vi "Draw 2D Plot.vi"(6 "Control Ref Queue":T1, 8 "error in (no error)":errorcluster, 10 "Multiplot Representation In":T2, 11 "2D Compass.lvclass in":refnum<class "2D Compass.lvclass">) -> (0 "error out":errorcluster, 2 "Multiplot Representation Out":T2, 3 "2D Compass.lvclass out":refnum<class "2D Compass.lvclass">)   [LabVIEW 2017, in "2D Compass.lvclass"]
uses:
  <vilib>/Math Plots/2D Math Plots/2D Compass/2D Compass/2D Compass.lvclass
  <vilib>/Math Plots/2D Math Plots/2D Plot/2D Plot/Typedef/Multiplot Representation.ctl
  <vilib>/Math Plots/2D Math Plots/2D Plot/2D Plot/Typedef/Plot Representation.ctl
  <vilib>/Math Plots/2D Math Plots/2D Plot/2D Plot/Typedef/Range Cluster.ctl
  <vilib>/Math Plots/2D Math Plots/2D Plot/Action String/2DMathPlot Ctrl Act Queue.ctl
  <vilib>/Math Plots/2D Math Plots/2D Plot/Action String/2DMathPlot Ctrl Act Cluster.ctl
  <vilib>/Math Plots/2D Math Plots/2D Plot/Action String/2DMathPlot State Class.ctl
  <vilib>/Math Plots/2D Math Plots/2D Compass/2D Compass/2D Compass.lvclass/2D Compass.ctl
  <vilib>/Math Plots/2D Math Plots/2D Plot/2D Plot/2D Plot.lvclass
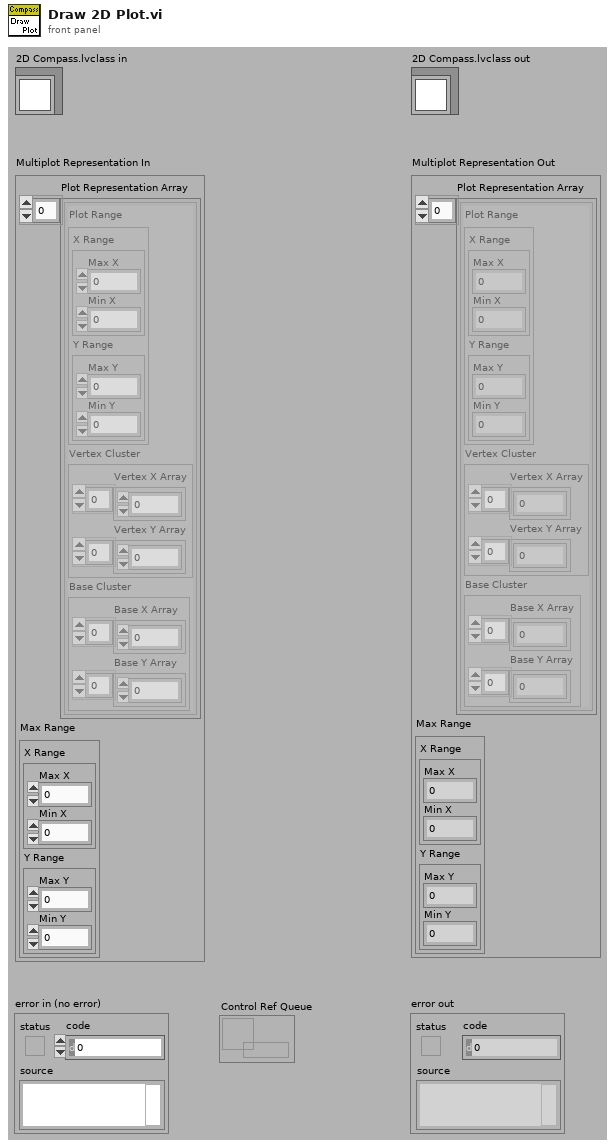
[diagram p1: front panel]
types:
  T1 = typedef "2DMathPlot Ctrl Act Queue.ctl" = refnum<queue>
  T2 = typedef "2D Plot.lvclass/Multiplot Representation.ctl" = cluster{"Plot Representation Array":T3[], "Max Range":T4}
  T3 = typedef "2D Plot.lvclass/Plot Representation.ctl" = cluster{"Plot Range":T4, "Vertex Cluster":cluster{"Vertex X Array":dbl[], "Vertex Y Array":dbl[]}, "Base Cluster":cluster{"Base X Array":dbl[], "Base Y Array":dbl[]}}
  T4 = typedef "2D Plot.lvclass/Range Cluster.ctl" = cluster{"X Range":cluster{"Max X":dbl, "Min X":dbl}, "Y Range":cluster{"Max Y":dbl, "Min Y":dbl}}
  T5 = typedef "2D Plot.lvclass/Plot Property Array.ctl" = T6[]
  T6 = typedef "2D Plot.lvclass/Plot Property.ctl" = cluster{"Bar Plot Style":u8, "DigitalLineStyle":u8, "TransitionLocation":u8, "Transition Type":u8, "Fill To":i16, "Fill/Pt. Color":u32, "Label Style":u8, "Line Style":u8, "Line Width":u8, "Plot Color":u32, "Plot Interpolation":u8, "Plot Name":string, "Point Style":u8, "Visible?":bool, "XScaleIdx":u32, "YScaleIdx":u32}
  T7 = typedef "2DMathPlot Ctrl Act Cluster.ctl" = cluster{"Plot Area Ref":refnum<vi>, "Z Axis Ref":refnum<vi>, "Legend Ref":refnum<vi>, "XControl Ref":refnum<vi>, "Facade Ref":refnum<vi>, "Display State Change Class":T8}
  T8 = typedef "2DMathPlot State Class.ctl" = enum16{"Update All (Undo)", "Update General", "Update Appearance", "Update Format", "Update Scale", "Update Marker", "Update Cursor", "None"}
  T9 = cluster{"Vertex X Array":dbl[], "Vertex Y Array":dbl[]}
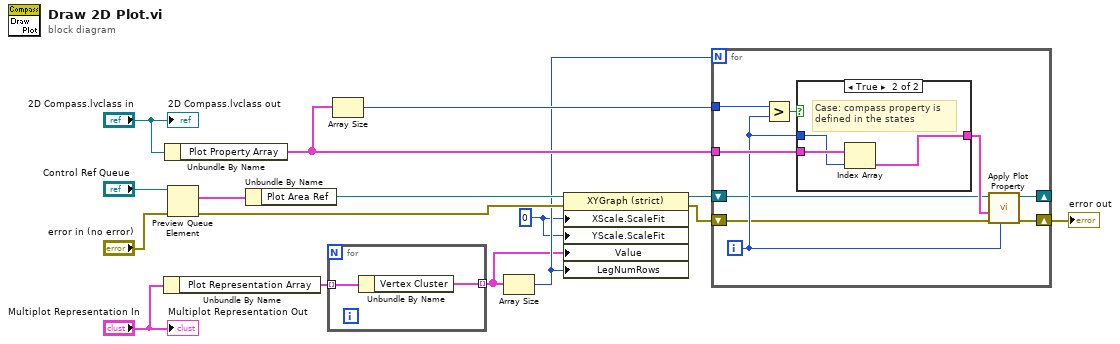
[diagram p0: block diagram]
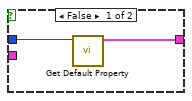
[diagram p2: hidden frame]
diagram:
  w1 = u8 0 ("X Scale.Scale Fit")
  n1 = Unbundle By Name("Multiplot Representation In") -> ("Plot Representation Array"=w11:T3[])
  n2 = Unbundle By Name("2D Compass.lvclass in") -> ("Plot Property Array"=w8:T5)
  n3 = Preview Queue Element(queue="Control Ref Queue", error in (no error)="error in (no error)") -> (element=w15:T7, error out=w10:errorcluster)  [unwired: 3 out]
  n4 = Unbundle By Name(w15) -> ("Plot Area Ref"=w9:refnum<vi>)
  n5 = for {
    tunnel: w11 -> [w18] mode=indexing
    tunnel: [w17] -> w2 mode=indexing
    n6 = Unbundle By Name(w18) -> ("Vertex Cluster"=w17:T9)
  }
  n7 = Array Size(array=w8) -> (size(s)=w5:i32)
  n8 = Array Size(array=w2) -> (size(s)=w4:i32)
  n9 = property class="XYGraph (strict)"(reference=w9, error in=w10, "XScale.ScaleFit"=w1, "YScale.ScaleFit"=w1, "Value"=w2, "LegNumRows"=w4) -> (reference out=w7:refnum<vi>, error out=w6:errorcluster)
  n10 = for {
    N: w4 -> [_]
    shift-right: [w25] -> _
    shift-left: w7 -> [w20]
    shift-right: [w26] -> w3
    shift-left: w6 -> [w19]
    tunnel: w8 -> [w27]
    tunnel: w5 -> [w24]
    i -> [w22]
    n11 = Greater?(x=w24, y=w22) -> (0:w23:bool)
    n12 = case shown="True" w23 {
      tunnel: w27 -> [_ w32]
      tunnel: w22 -> [w28 w31]
      tunnel: [w29 w30] -> w21
      frame False {
        n13 = call <vilib>:"Get Default Property.vi"("Index"=w28) -> ("Temporary Property"=w29:T6)  [unwired: 4 in, 6 out]
      }
      frame True {
        # "Case: compass property is \ndefined in the states"
        n14 = Index Array(array=w32, index=w31) -> (element=w30:T6)
      }
    }
    n15 = call <vilib>:"Apply Plot Property.vi"("Plot ID"=w22, "error in (no error)"=w19, "Plot Property"=w21, "Polar Area Ref In"=w20) -> ("error out"=w26:errorcluster, "Polar Area Ref Out"=w25:refnum<vi>)  [unwired: 1 in, 5 out]
  }
  "error out" <- w3
  "2D Compass.lvclass out" <- "2D Compass.lvclass in"
  "Multiplot Representation Out" <- "Multiplot Representation In"
